vi "DPT Panel Init Dry Flow Meter.vi"(11 "Error In":errorcluster) -> (6 "Heat Val.":dbl, 8 "BTUF3":string[][](array[string]), 15 "Error Out":errorcluster)   [LabVIEW 2016]
uses:
  Utility/Custom Pallet Controls/Custom Pallet DBL.ctl
  Utility/Custom Pallet Controls/Custom Pallet Forward.ctl
panel:
  in  "File Setup OK":T1
  in  "Today's Calorimeter\nReading (BTU/ft3)":T2 format="%.2f"
  in  "Gas Type":string(combo)="Natural Gas"
  in  "lower limit":dbl=500.0
  in  "upper limit":dbl=5000.0
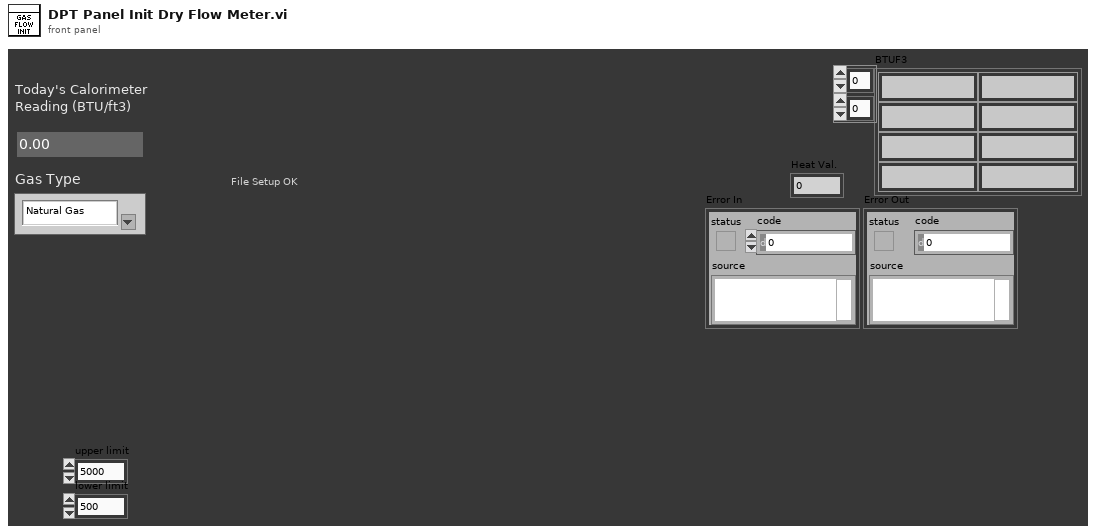
[diagram p1: front panel]
types:
  T1 = typedef "Custom Pallet Forward.ctl" = bool
  T2 = typedef "Custom Pallet DBL.ctl" = dbl
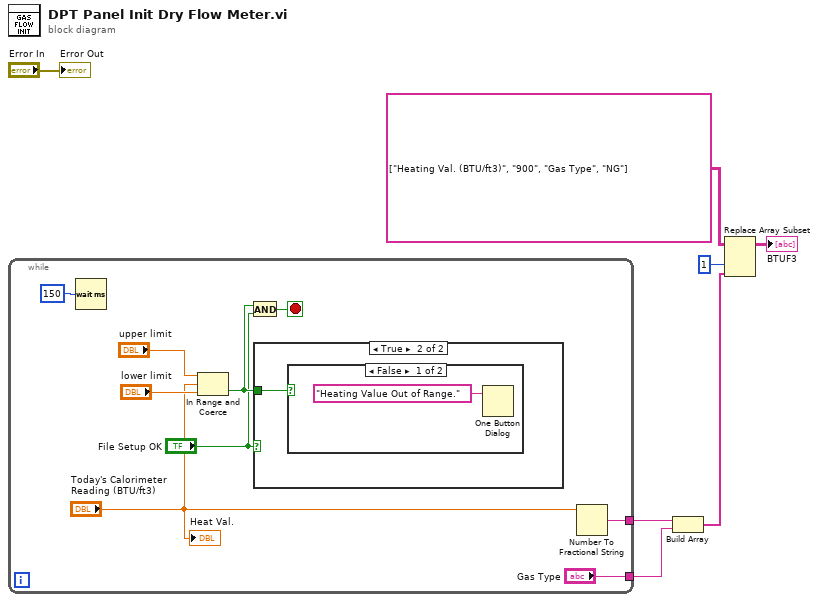
[diagram p0: block diagram]
diagram:
  n1 = while {
    tunnel: [w10] -> w4
    tunnel: ["Gas Type"] -> w2
    stop <- w13 stop-if-true
    n2 = Wait (ms)(milliseconds to wait=u32 150) -> ()  [unwired: 1 out]
    n3 = In Range and Coerce(upper limit="upper limit", x="Today's Calorimeter\nReading (BTU/ft3)", lower limit="lower limit") -> (In Range?=w12:bool)  [unwired: 1 out]
    n4 = And(x=w12, y="File Setup OK") -> (x .and. y?=w13:T1)
    n5 = case shown="True" "File Setup OK" {
      tunnel: w12 -> [_ w17]
      frame False {
      }
      frame True {
        n6 = case shown="False" w17 {
          frame False {
            n7 = One Button Dialog(message="Heating Value Out of Range.") -> ()  [unwired: 1 in, 1 out]
          }
          frame True {
          }
        }
      }
    }
    n8 = Number To Fractional String(number="Today's Calorimeter\nReading (BTU/ft3)") -> (F-format string=w10:string)  [unwired: 3 in]
    "Heat Val." <- "Today's Calorimeter\nReading (BTU/ft3)"
  }
  n9 = Build Array(w4, w2) -> (w3:string[])
  n10 = Replace Array Subset(array=string[][] [["Heating Val. (BTU/ft3)", "900"], ["Gas Type", "NG"]] ("appended array"), new element=w3, index (col)=1 ("disabled index (col)")) -> (→"BTUF3":string[][])  [unwired: 1 in]
  "Error Out" <- "Error In"
